vi "SubVI_ArcadeTester.vi"(10 "forward input":dbl(slide) scale=-1.0..1.0, 11 "left input":dbl(slide) scale=1.0..-1.0) -> (2 "Right Predicted":dbl(slide) scale=-18000.0..18000.0, 3 "Left Predicted":dbl(slide) scale=-18000.0..18000.0)   [LabVIEW 2017]
panel:
  in  "Scale":dbl=36000.0 format="%#_13g"
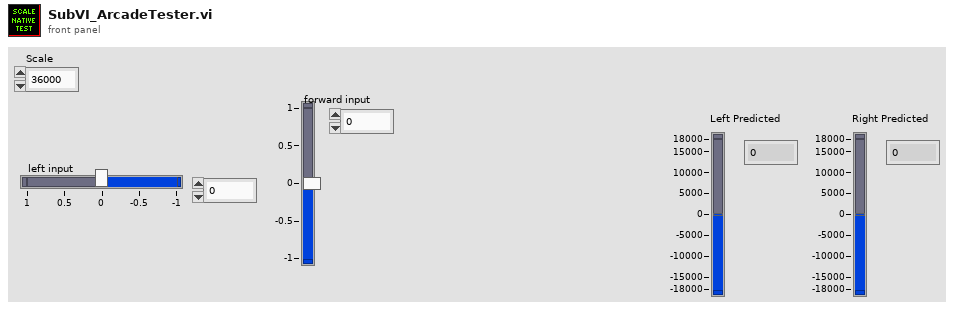
[diagram p1: front panel]
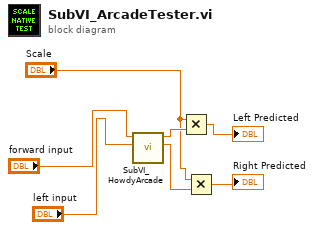
[diagram p0: block diagram]
diagram:
  n1 = call "SubVI_HowdyArcade.vi"("X axis value"="left input", "Y axis value"="forward input") -> ("right"=w4:dbl, "left"=w5:dbl)  [unwired: 8 in]
  n2 = Multiply(x="Scale", y=w5) -> (x*y=→"Left Predicted":dbl)
  n3 = Multiply(x="Scale", y=w4) -> (x*y=→"Right Predicted":dbl)
